vi "Set Turbo Valve.vi"(8 "error in (no error)":errorcluster, 9 "Interlock Chain.lvclass":refnum<class "Interlock Chain.lvclass">, 10 "Open? (False)":bool, 11 "Turbo in":refnum<class "Turbo.lvclass">) -> (0 "error out":errorcluster, 3 "Turbo out":refnum<class "Turbo.lvclass">)   [LabVIEW 2015, in "cRIO-Carbondioxide.lvlib" / "CO2-Actor.lvlib" / "Turbo.lvclass"]
uses:
  Turbo.lvclass
  Interlocks/Interlock Chain/Interlock Chain.lvclass
  <vilib>/ActorFramework/Actor/Actor.lvclass/Actor.ctl
  <vilib>/ActorFramework/Message Enqueuer/Message Enqueuer.lvclass/Message Enqueuer.ctl
  Turbo.lvclass/Turbo.ctl
  Valve Messages/Write Bit Field Msg/Write Bit Field Msg.lvclass/Write Bit Field Msg.ctl
  <vilib>/ActorFramework/Actor/Read Self Enqueuer.vi
  <vilib>/ActorFramework/Message Enqueuer/Enqueue.vi
  <vilib>/ActorFramework/Message Enqueuer/Init from Existing Queue.vi
  <vilib>/ActorFramework/Message Priority Queue/Priority Enqueue.vi
  <vilib>/ActorFramework/Actor/Actor.lvclass
  <vilib>/ActorFramework/Message Enqueuer/Message Enqueuer.lvclass
  Valve Messages/Write Bit Field Msg/Write Bit Field Msg.lvclass
  CO2 Actor/CO2 Actor.lvclass
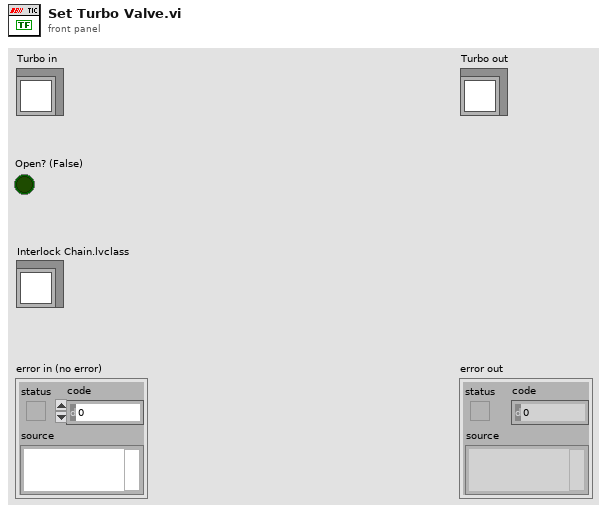
[diagram p1: front panel]
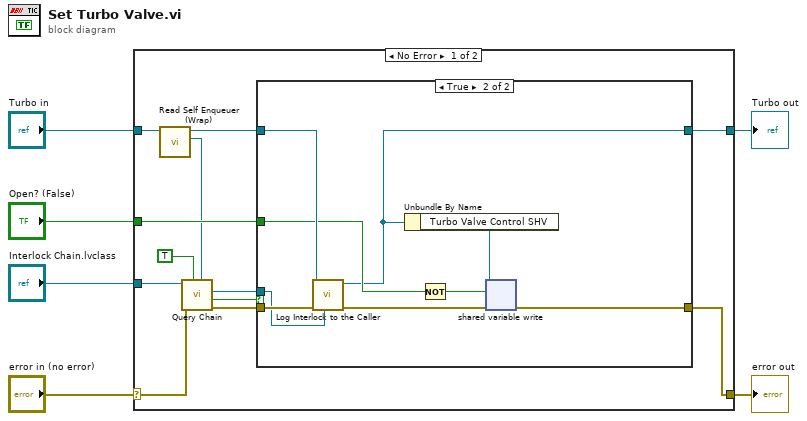
[diagram p0: block diagram]
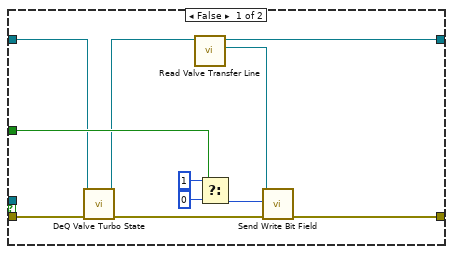
[diagram p2: hidden frame]
diagram:
  n1 = case shown="No Error" "error in (no error)" {
    selector: "error in (no error)" -> [w17 w40]
    tunnel: [w10 w40] -> w5
    tunnel: [w12 w39] -> w3
    tunnel: "Turbo in" -> [w9 w39]
    tunnel: "Open? (False)" -> [w13 _]
    tunnel: "Interlock Chain.lvclass" -> [w18 _]
    frame No Error {
      n2 = call "Read Self Enqueuer (Wrap).vi"("CO2 Actor in"=w9) -> ("Actor Framework:Message Enqueuer"=w7:refnum<class "Message Enqueuer.lvclass">, "CO2 Actor out"=w8:refnum<class "Turbo.lvclass">)  [unwired: 9 in]
      n3 = call "Query Chain.vi"("Caller Enqueuer"=w7, "Close Connections (F)"=TRUE, "error in (no error)"=w17, "Interlock Chain"=w18) -> ("error out"=w15:errorcluster, "Interlock?"=w11:bool, "Interlock out"=w14:refnum<class "Interlock.lvclass">)  [unwired: 2 in, 3 out]
      n4 = case shown="True" w11 {
        tunnel: w15 -> [w22 w38]
        tunnel: w14 -> [_ w37]
        tunnel: w8 -> [w20 w36]
        tunnel: [w23 w30] -> w12
        tunnel: w13 -> [w26 w33]
        tunnel: [w24 w31] -> w10
        frame False {
          n5 = call "DeQ Valve Turbo State.vi"("error in (no error)"=w22, "Turbo in"=w20) -> ("error out"=w21:errorcluster, "Turbo out"=w19:refnum<class "Turbo.lvclass">)  [unwired: 6 in, 2 out]
          n6 = call "Read Valve Transfer Line.vi"("Turbo in"=w19) -> ("Actor Framework:Message Enqueuer"=w25:refnum<class "Message Enqueuer.lvclass">, "Turbo out"=w23:refnum<class "Turbo.lvclass">)  [unwired: 9 in]
          n7 = Select(t=u16 1, s=w26, f=u16 0 ("Bit Field")) -> (s? t:f=w27:u16)
          n8 = call "Send Write Bit Field.vi"("error in (no error)"=w21, "Bit Field"=w27, "Message Enqueuer"=w25) -> ("error out"=w24:errorcluster)  [unwired: 5 in, 3 out]
        }
        frame True {
          n9 = call-dynamic "Log Interlock to the Caller.vi"("Interlock in"=w37, "error in (no error)"=w38, "CO2 Actor in"=w36) -> ("error out"=w35:errorcluster, "CO2 Actor out"=w30:refnum<class "Turbo.lvclass">)  [unwired: 7 in]
          n10 = Unbundle By Name(w30) -> ("Turbo Valve Control SHV"=w34:refnum<k21>)
          n11 = Not(x=w33) -> (.not. x?=w32:bool)
          n12 = shared-variable-write(w34, w35, w32) -> (w31:errorcluster)  [unwired: 1 out]
        }
      }
    }
    frame Error {
    }
  }
  "error out" <- w5
  "Turbo out" <- w3
